vi "Habid_2-D_Histogram_Alpha.vi"() -> ()   [LabVIEW 2009]
uses:
  <vilib>/Utility/file.llb/Write To Spreadsheet File (DBL).vi
  <vilib>/Analysis/3filter.llb/Butterworth Filter (DBL).vi
  <vilib>/Analysis/NI_AALBase.lvlib
  <vilib>/Analysis/NI_AALPro.lvlib
panel:
  in  "Save 2-D":bool
  in  "Result File Dir 2":path
  in  "Result File Name 2":string="2D_Histogram.txt"
  in  "Piezo Factor":dbl=0.88881
  in  "High Voltage Gain":dbl=0.796905
  out "Total 2D Histogram":dbl[][](graph)
  out "Individual 2D Histogram":dbl[][](graph)
  out "After I(t)":cluster{dbl, dbl, "Filtered X":dbl[]}(graph)
  out "Before I(t)":cluster{dbl, "SamplingTime":dbl, "Data":ext[]}(graph)
  in  "start path":path=path "J:/data"
  out "NormAC":dbl[](array[numeric])
  in  "Save Curve?":bool
  out "CurrentFileName":string
  in  "Result File Name":string="1D_Histogram.txt"
  in  "Result File Dir":path
  in  "Save 1-D":bool
  out "SelectedCurves":i32
  out "CurvesInHistogram":bool[](array[boolean])
  in  "Bias(V)":dbl=0.4
  in  "Preamp(A/V)":dbl=1e-08
  out "1-D Histogram":cluster{dbl[], dbl[]}(graph)
  in  "Beta Cutoff max":dbl=20.0
  in  "Beta Cutoff min":dbl
  in  "1-D Histogram?":bool
  in  "Continuous?":bool
  in  "Add Histogram?":bool
  in  "Beta bins":i32=400
  in  "Beta max":dbl=20.0
  in  "Beta min":dbl
  in  "log(I) bins":i32=400
  in  "log(I) max":dbl=1.0
  in  "log(I) min":dbl=-3.0
  in  "+/-":bool=TRUE
  out "DcData":dbl[](array[numeric])
  out "Beta":dbl[](array[numeric])
  out "DcDataLog":dbl[](array[numeric])
  out "TotalCurves":i32
  out "CurrentCurve":i32
  in  "Next Curve":bool
  in  "Previous Curve":bool
  out "AC I(t)":T1(graph)
  in  "Piezo Sensitivity (nm/V)":dbl=3.89
  in  "Z-mod Amp (V)":dbl=0.0257
  in  "Gac/Gdc":dbl=1.43369
  in  "low cutoff freq: fl":u32=1200
  in  "high cutoff freq: fh":u32=2800
  out "DC I(t)":T2(graph)
  in  "DC cutoff freq":i32=600
  out "Original I(t)":cluster{dbl, "SamplingTime":dbl, "Data":ext[]}(graph)
  out "DataBuffer":dbl[](array[numeric])
  out "Sampling Freq":dbl
  out "Sampling Time":dbl
  out "TimeLine":dbl[](array[numeric])
  in  "stop":bool
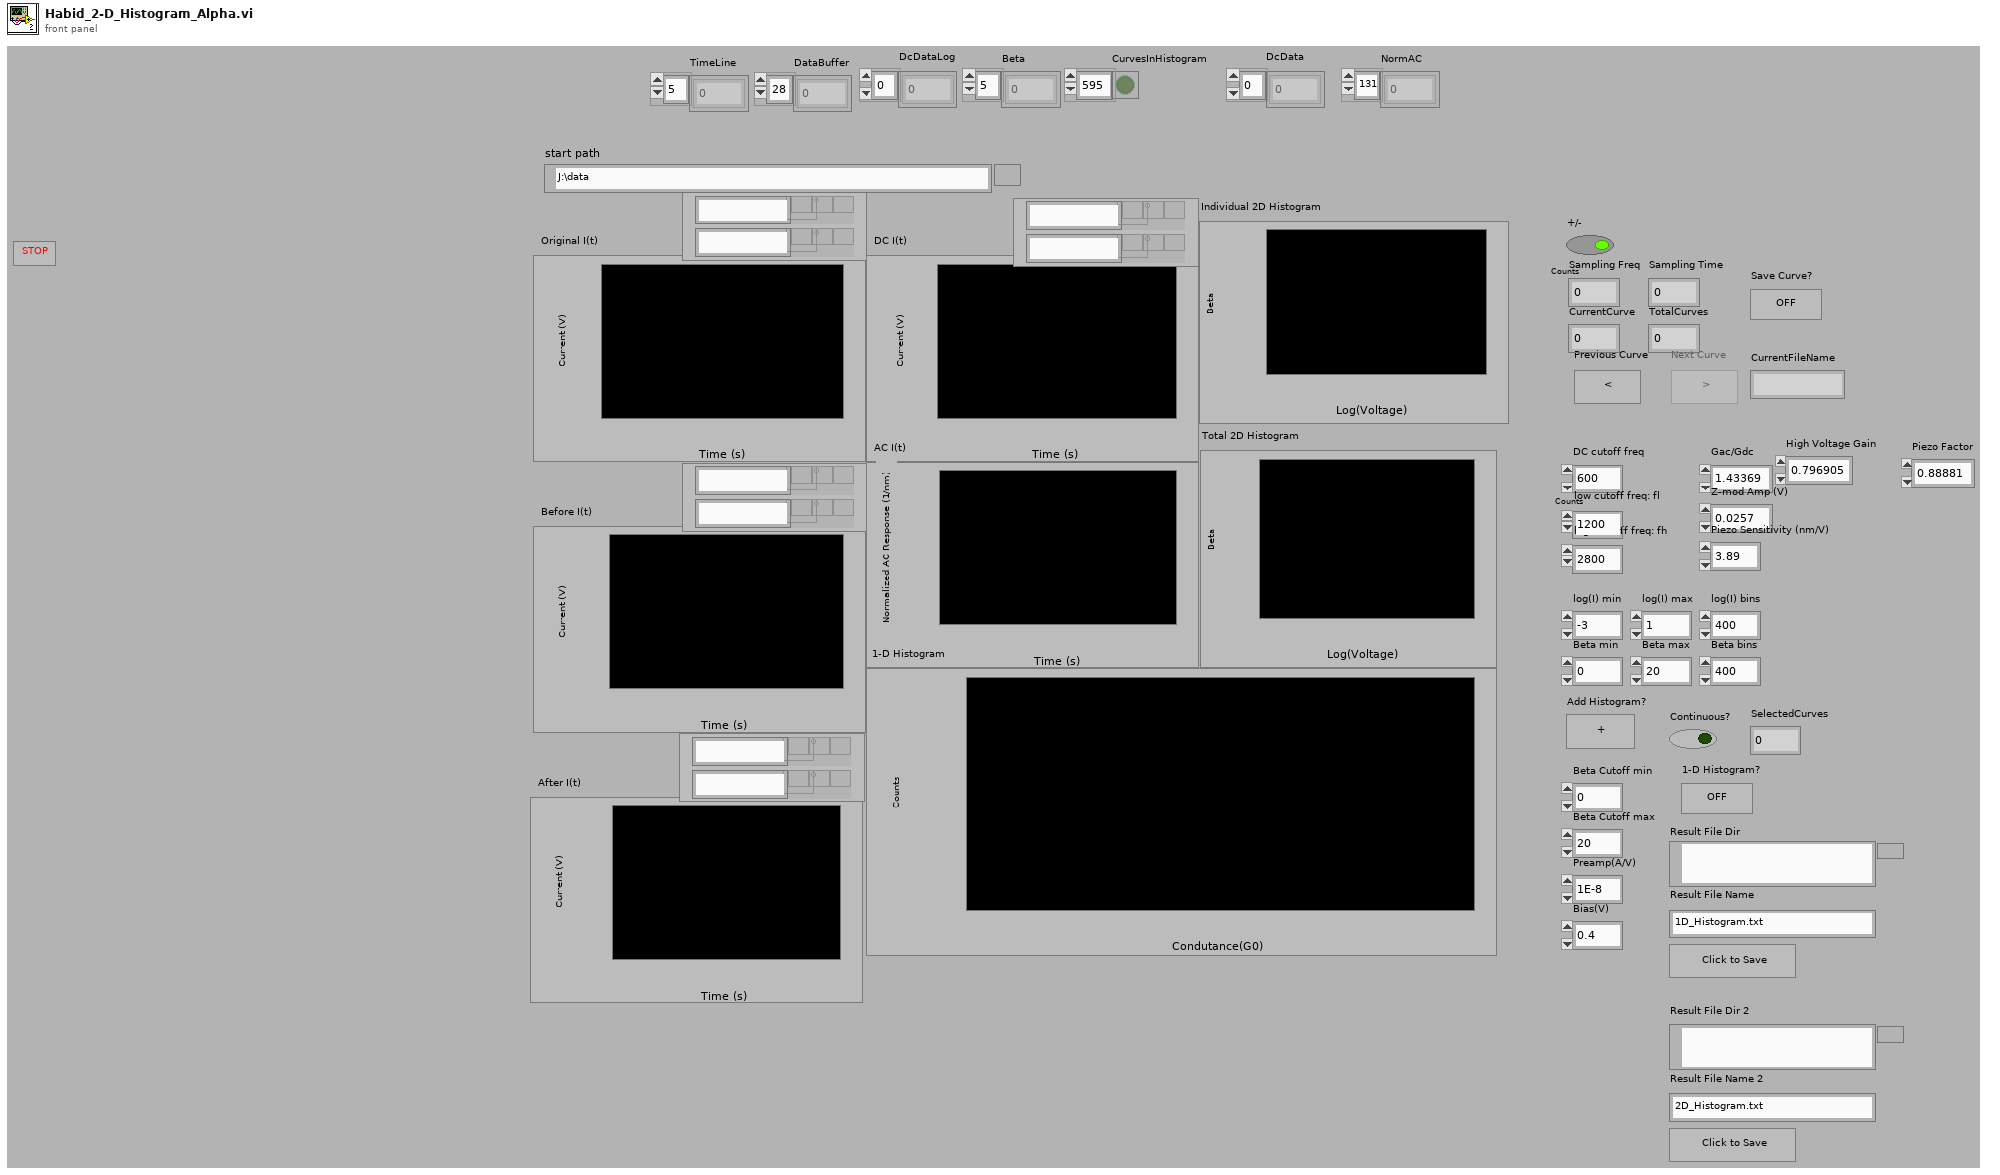
[diagram p1: front panel]
types:
  T1 = cluster{"Start Time":dbl, "Sampling Time":dbl, dbl[][]}
  T2 = cluster{dbl, "SamplingTime":dbl, "Filtered X":dbl[]}
  T3 = enum32{"Lowpass", "Highpass", "Bandpass", "Bandstop"}
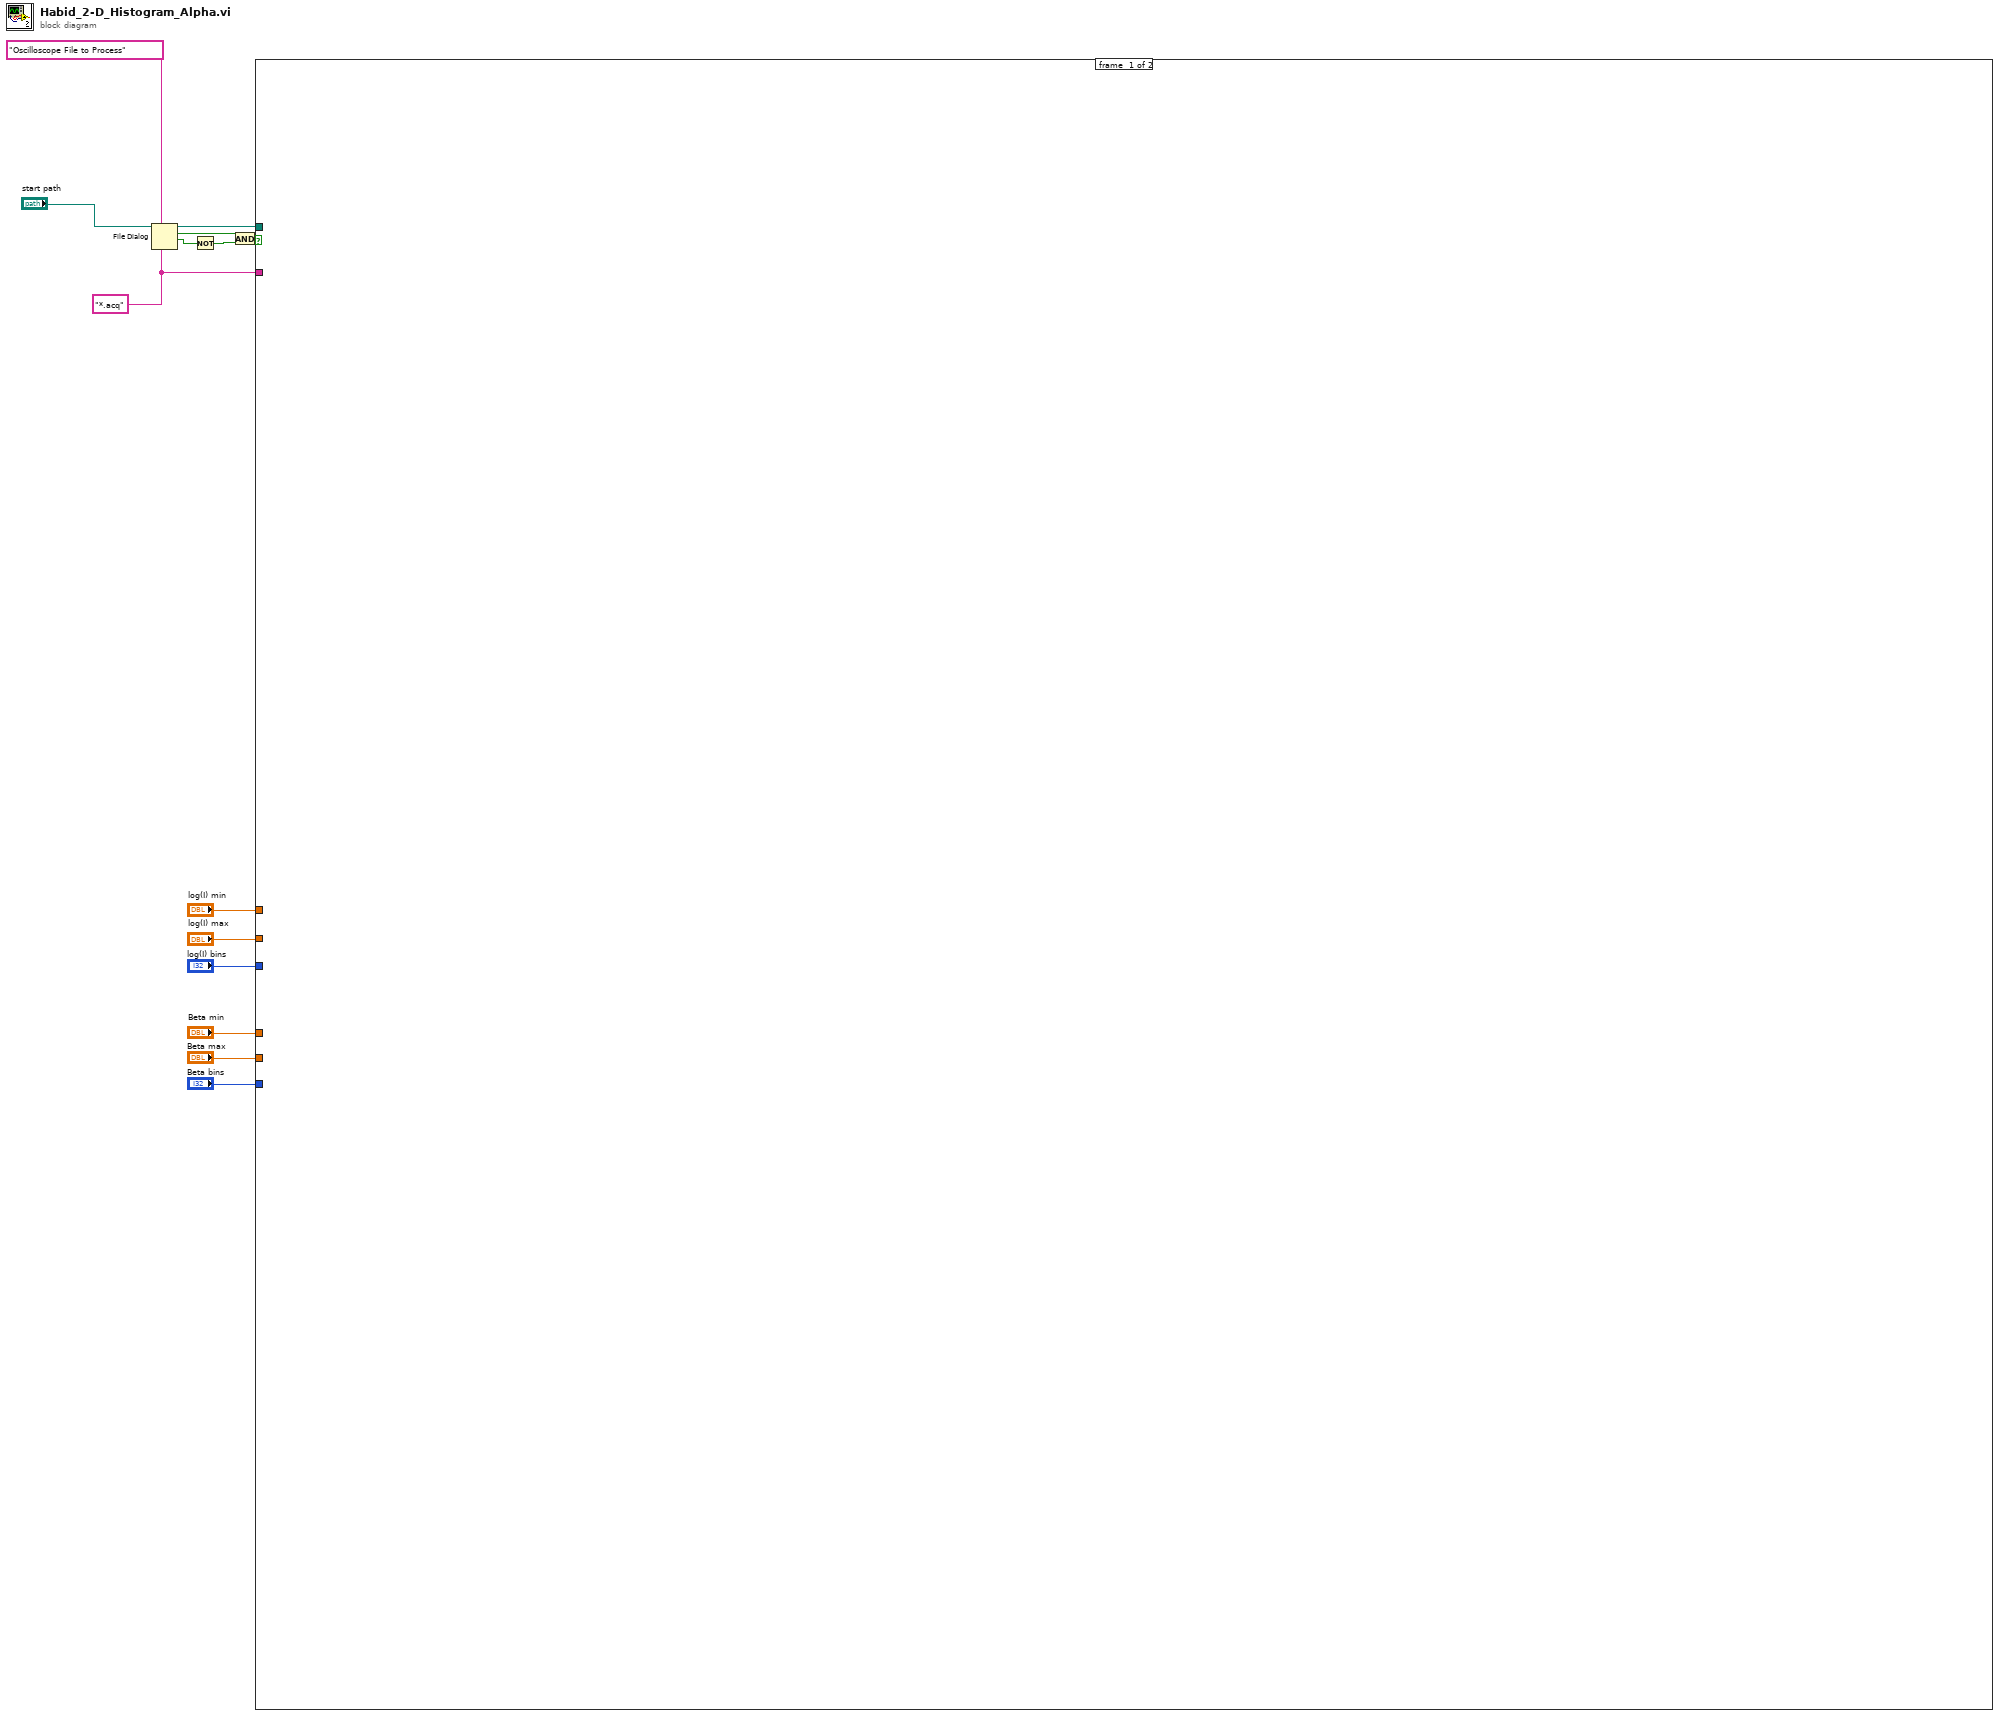
[diagram p0: block diagram]
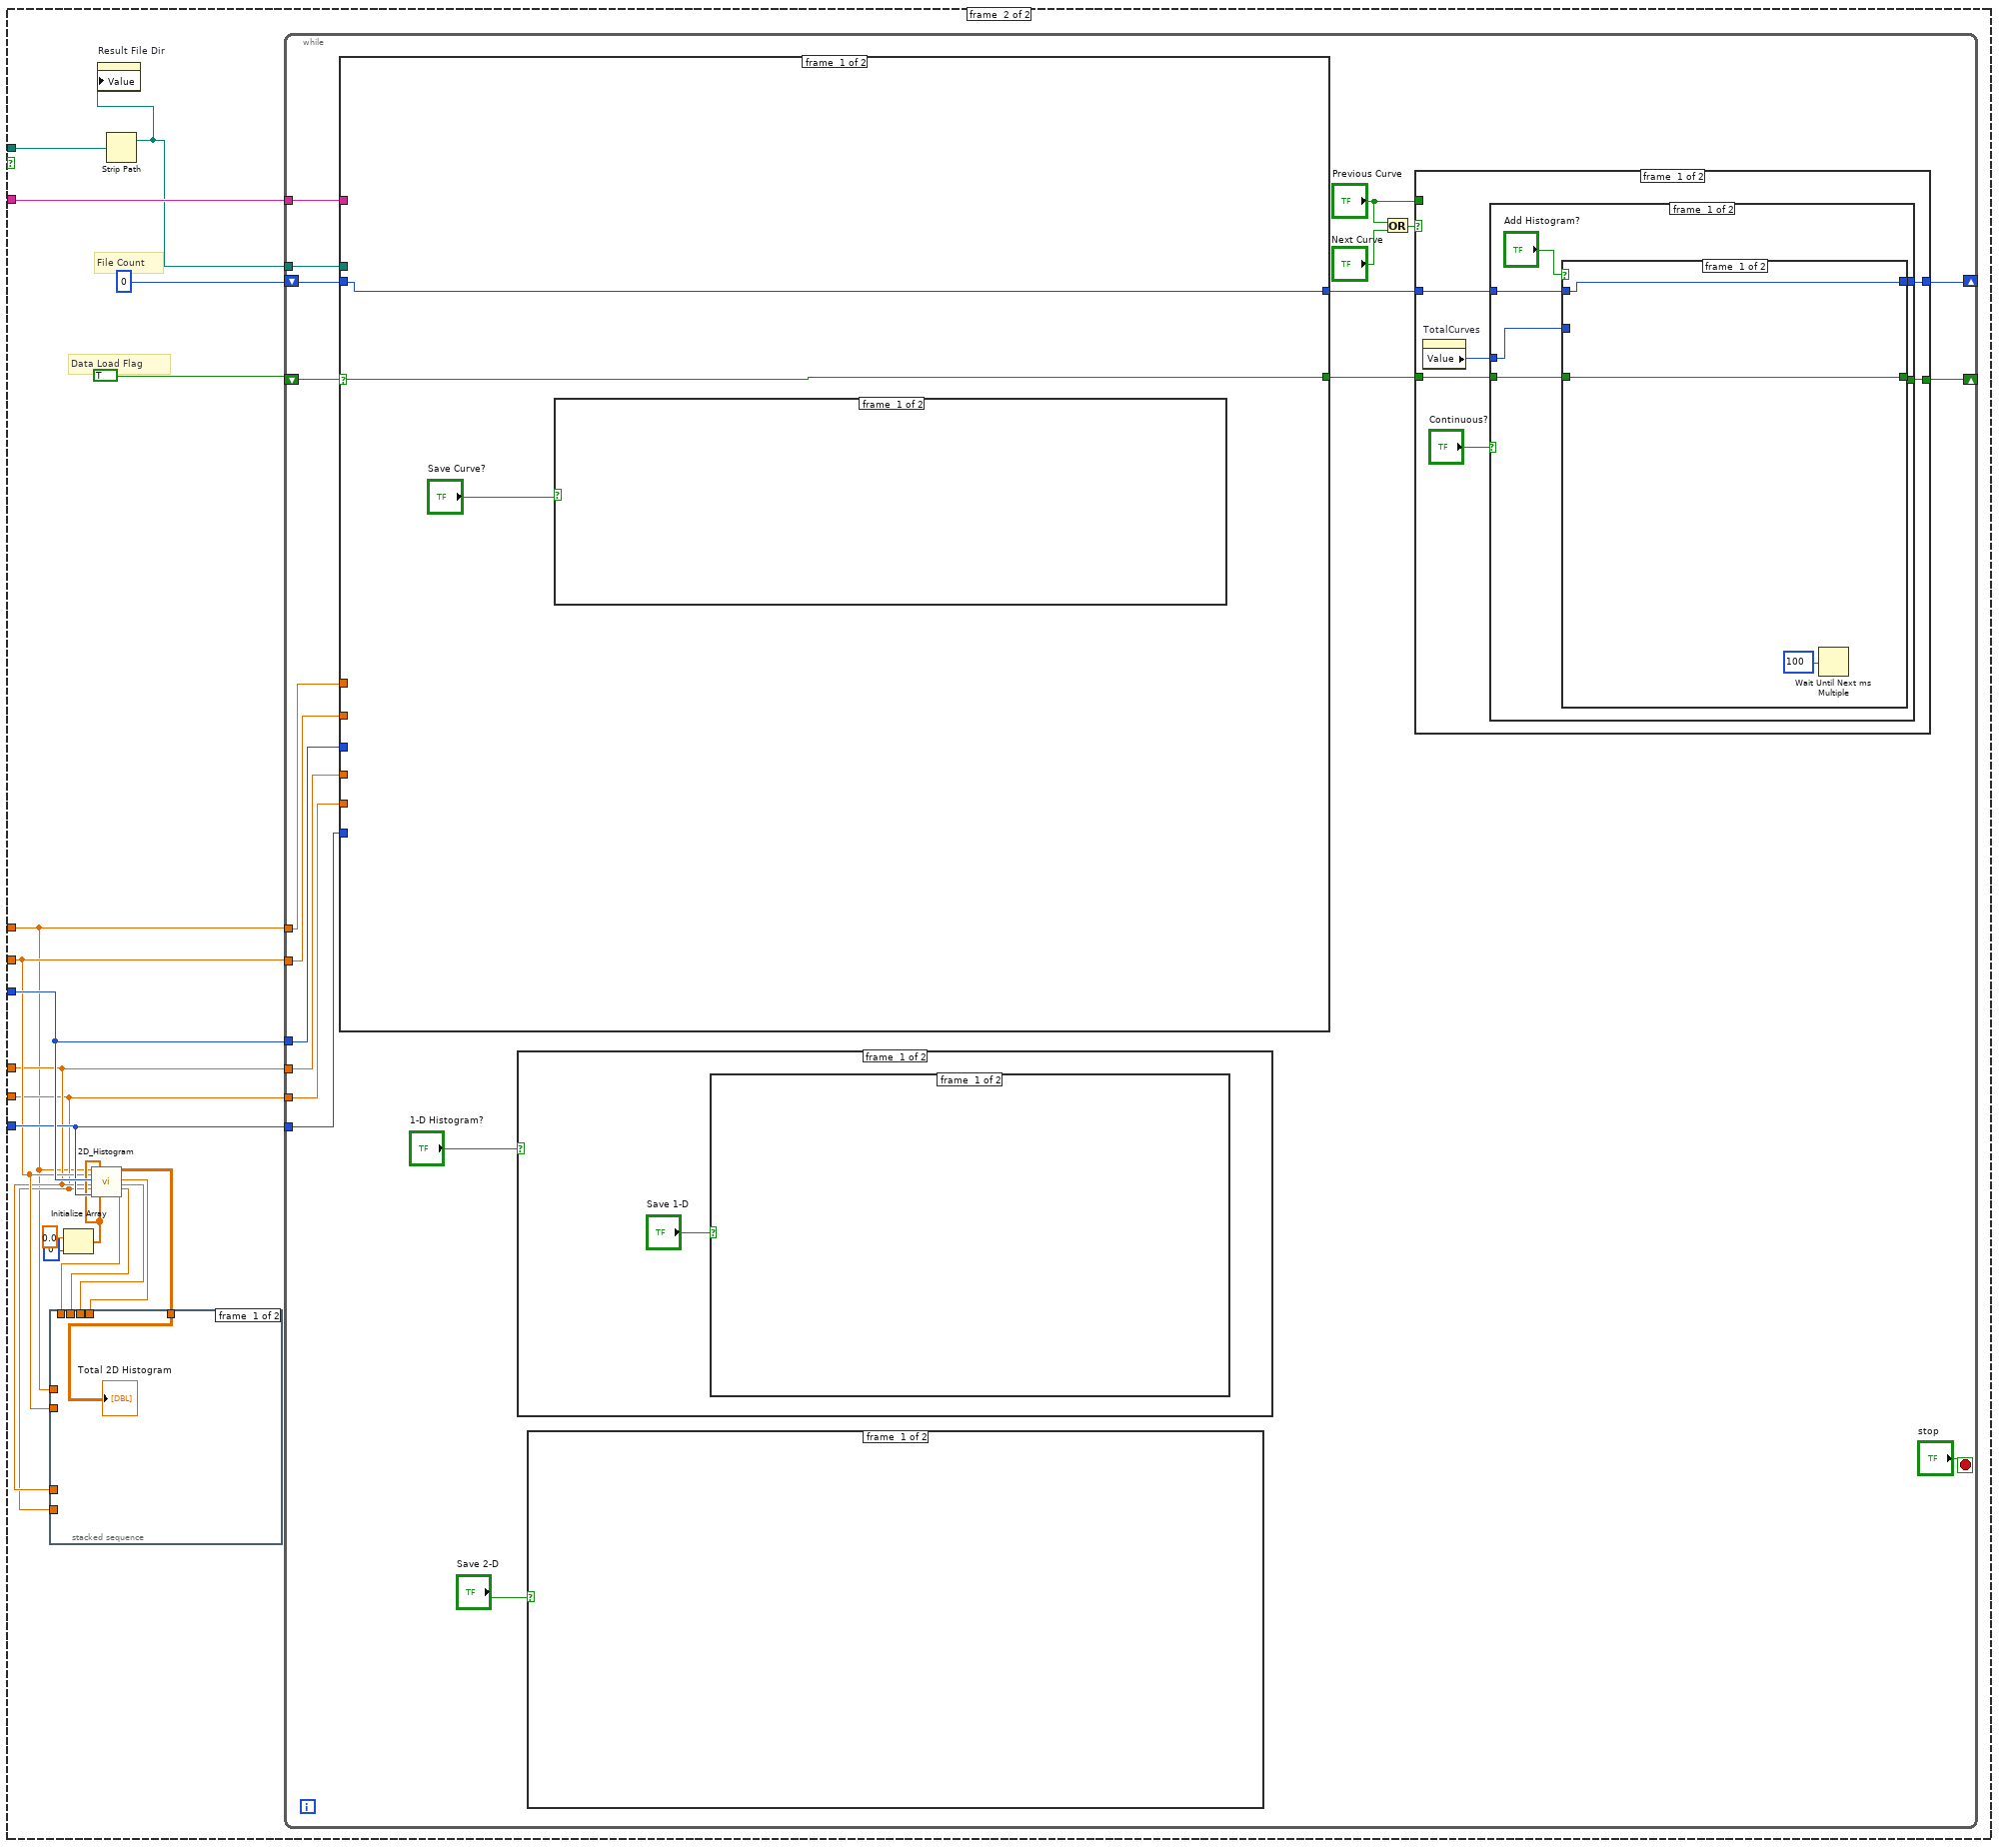
[diagram p2: hidden frame]
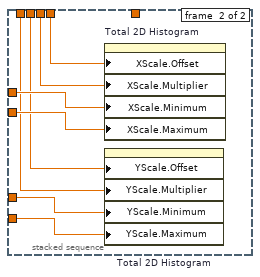
[diagram p3: hidden frame]
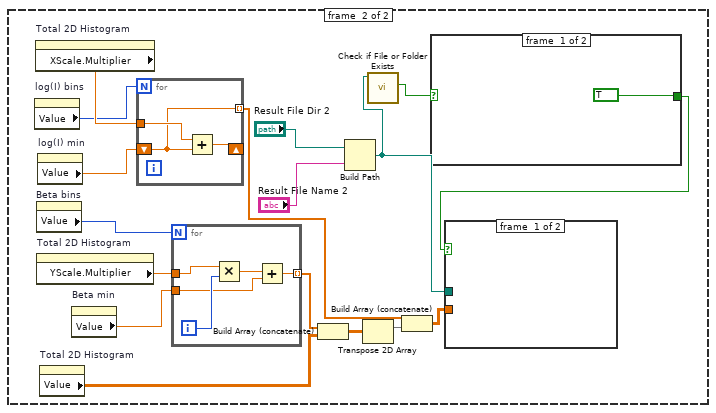
[diagram p4: hidden frame]
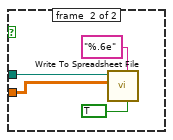
[diagram p5: hidden frame]
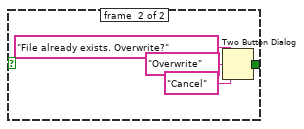
[diagram p6: hidden frame]
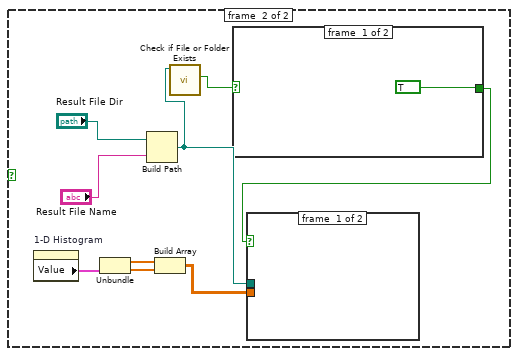
[diagram p7: hidden frame]
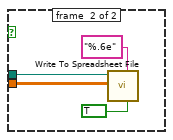
[diagram p8: hidden frame]
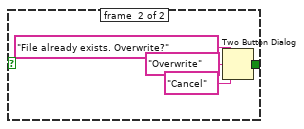
[diagram p9: hidden frame]
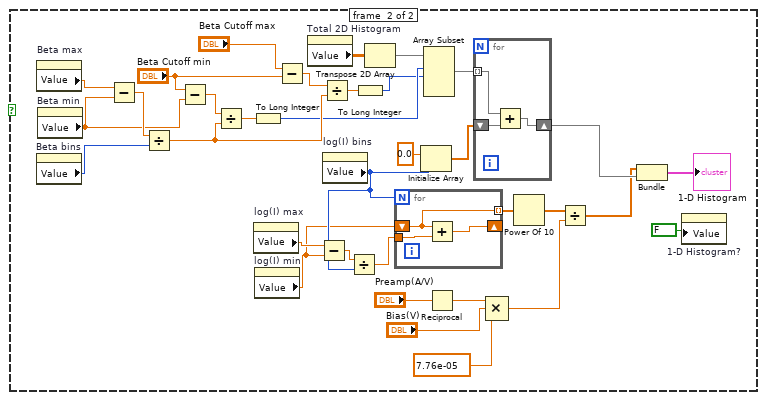
[diagram p10: hidden frame]
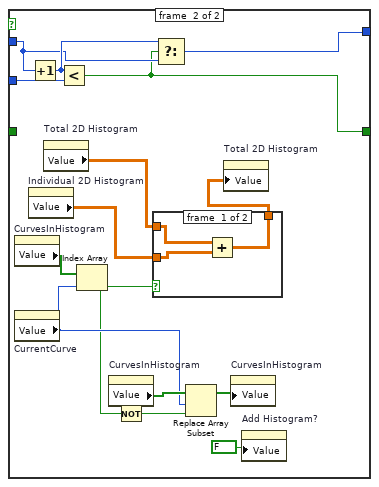
[diagram p11: hidden frame]
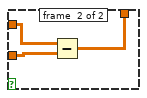
[diagram p12: hidden frame]
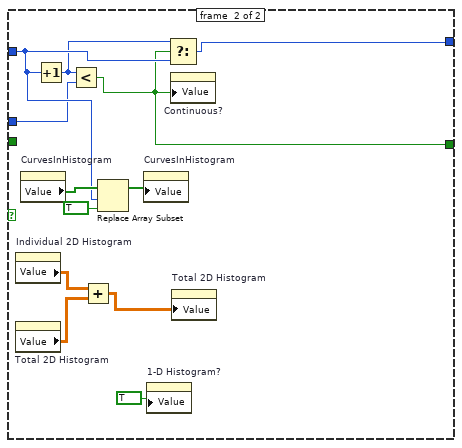
[diagram p13: hidden frame]
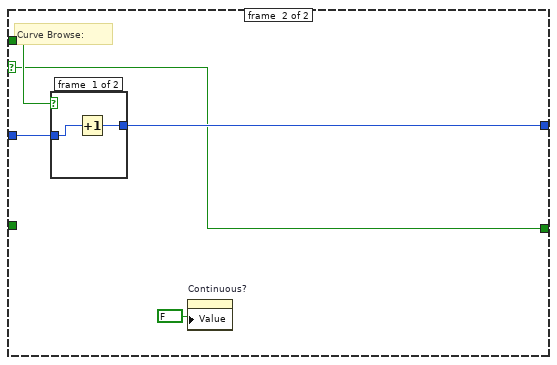
[diagram p14: hidden frame]
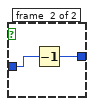
[diagram p15: hidden frame]
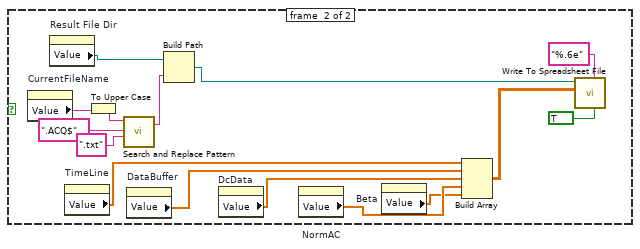
[diagram p16: hidden frame]
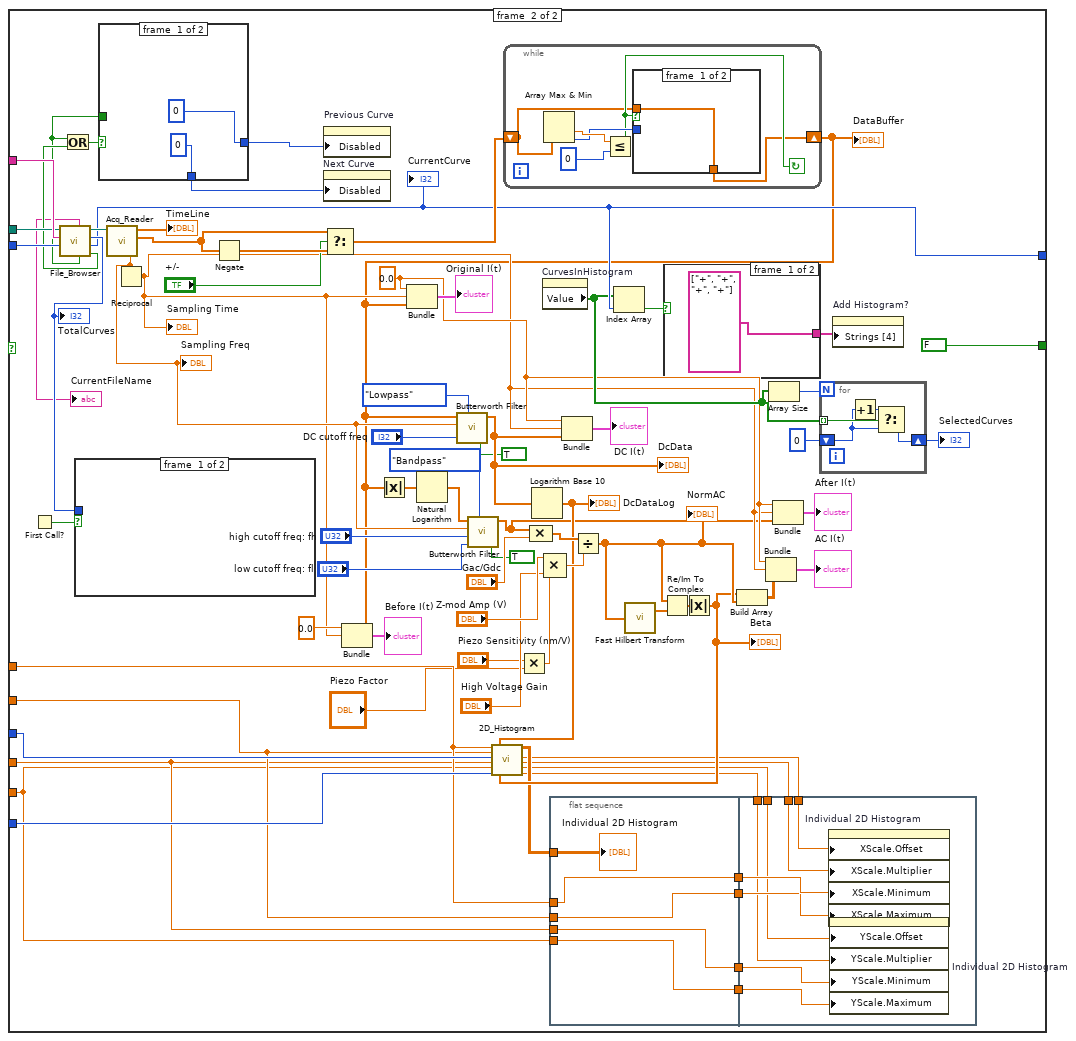
[diagram p17: hidden frame]
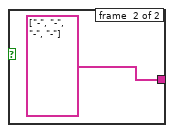
[diagram p18: hidden frame]
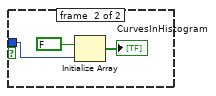
[diagram p19: hidden frame]
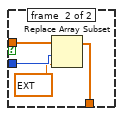
[diagram p20: hidden frame]
diagram:
  w7 = "*.acq" ("pattern (all files)")
  n1 = File Dialog(6:w7, 7:"Oscilloscope File to Process", 11:"start path") -> (1:w11:bool, 2:w13:bool, 3:w8:path)  [unwired: 4 in, 1 out]
  n2 = Not(x=w11) -> (.not. x?=w12:bool)
  n3 = And(x=w13, y=w12) -> (x .and. y?=w9:bool)
  n4 = case shown="True" w9 {
    tunnel: w8 -> [_ w33]
    tunnel: w7 -> [_ w31]
    tunnel: "log(I) min" -> [_ w15]
    tunnel: "log(I) max" -> [_ w18]
    tunnel: "log(I) bins" -> [_ w29]
    tunnel: "Beta min" -> [_ w17]
    tunnel: "Beta max" -> [_ w16]
    tunnel: "Beta bins" -> [_ w28]
    frame #0 {
    }
    frame #1 {
      # "File Count"
      # "Data Load Flag"
      n5 = Initialize Array(0.0 ("element"), 0 ("dimension size")) -> (w20:dbl[])
      n6 = call "2D_Histogram.vi"("X min"=w15, "X max"=w18, "X bins"=w29, "Y min"=w17, "Y max"=w16, "Y bins"=w28, "X"=w20, "Y"=w20) -> ("X-Y 2-D Histogram"=w27:dbl[][], "Xoffset"=w26:dbl, "Xmultiplier"=w25:dbl, "Yoffset"=w24:dbl, "Ymultiplier"=w23:dbl)  [unwired: 7 in]
      n7 = stacked-sequence {
        tunnel: w27 -> [w34 _]
        tunnel: w25 -> [_ w41]
        tunnel: w23 -> [_ w37]
        tunnel: w26 -> [_ w42]
        tunnel: w24 -> [_ w38]
        tunnel: w15 -> [_ w40]
        tunnel: w18 -> [_ w39]
        tunnel: w17 -> [_ w36]
        tunnel: w16 -> [_ w35]
        frame #0 {
          "Total 2D Histogram" <- w34
        }
        frame #1 {
          n8 = property on="Total 2D Histogram" class="IntGraph (strict)"("XScale.Offset"=w42, "XScale.Multiplier"=w41, "XScale.Minimum"=w40, "XScale.Maximum"=w39) -> ()  [unwired: 2 in, 2 out]
          n9 = property on="Total 2D Histogram" class="IntGraph (strict)"("YScale.Offset"=w38, "YScale.Multiplier"=w37, "YScale.Minimum"=w36, "YScale.Maximum"=w35) -> ()  [unwired: 2 in, 2 out]
        }
      }
      n10 = Strip Path(path=w33) -> (stripped path=w19:path)  [unwired: 1 out]
      n11 = property on="Result File Dir" class="Path"("Value"=w19) -> ()  [unwired: 2 in, 2 out]
      n12 = while {
        shift-right: [w45] -> _
        shift-left: TRUE ("DataReload") -> [w61]
        tunnel: w31 -> [w60]
        tunnel: w19 -> [w59]
        shift-right: [w46] -> _
        shift-left: 0 -> [w58]
        tunnel: w15 -> [w55]
        tunnel: w18 -> [w54]
        tunnel: w29 -> [w53]
        tunnel: w17 -> [w52]
        tunnel: w16 -> [w51]
        tunnel: w28 -> [w50]
        stop <- "stop" stop-if-true
        n13 = case shown="True" w61 {
          selector: w61 -> [w215 _]
          tunnel: w60 -> [_ w305]
          tunnel: w59 -> [_ w304]
          tunnel: w58 -> [w214 w303]
          tunnel: [w215 FALSE] -> w57
          tunnel: [w214 w259] -> w56
          tunnel: w55 -> [_ w254]
          tunnel: w54 -> [_ w253]
          tunnel: w53 -> [_ w265]
          tunnel: w52 -> [_ w252]
          tunnel: w51 -> [_ w251]
          tunnel: w50 -> [_ w264]
          frame #0 {
            n14 = case shown="True" "Save Curve?" {
              frame #0 {
              }
              frame #1 {
                n15 = property on="CurrentFileName" class="Str"() -> ("Value"=w226:string)  [unwired: 2 in, 2 out]
                n16 = property on="Result File Dir" class="Path"() -> ("Value"=w230:path)  [unwired: 2 in, 2 out]
                n17 = property on="TimeLine" class="Arr (strict)"() -> ("Value"=w220:dbl[])  [unwired: 2 in, 2 out]
                n18 = To Upper Case(1:w226) -> (0:w227:string)
                n19 = call <vilib>:"Search and Replace Pattern.vi"("string"=w227, "regular expression (\"\")"=".ACQ$" ("regular expression (\"\")"), "replace string (\"\")"=".txt" ("replace string (\"\")")) -> ("result string"=w225:string)  [unwired: 2 in, 1 out]
                n20 = property on="DataBuffer" class="Arr (strict)"() -> ("Value"=w219:dbl[])  [unwired: 2 in, 2 out]
                n21 = Build Path(base path=w230, name or relative path=w225) -> (appended path=w222:path)
                n22 = property on="DcData" class="Arr (strict)"() -> ("Value"=w218:dbl[])  [unwired: 2 in, 2 out]
                n23 = property on="NormAC" class="Arr (strict)"() -> ("Value"=w217:dbl[])  [unwired: 2 in, 2 out]
                n24 = property on="Beta" class="Arr (strict)"() -> ("Value"=w216:dbl[])  [unwired: 2 in, 2 out]
                n25 = Build Array(w220, w219, w218, w217, w216) -> (w221:dbl[][])
                n26 = call-poly <vilib>:"Write To Spreadsheet File.vi"("transpose? (no:F)"=TRUE, "format (%.3f)"="%.6e", "2D data"=w221, "file path (dialog if empty)"=w222) -> ()  [unwired: 4 in, 1 out]
              }
            }
          }
          frame #1 {
            w240 = 0.0
            n27 = First Call?() -> (First Call?: T/F=w263:bool)
            n28 = call "File_Browser.vi"("FileIndexIn"=w303, "FileExt"=w305, "FolderPath"=w304) -> ("Last?"=w280:bool, "FileIndexOut"=w259:i32, "FileTotal"=w262:i32, "FullFilePath"=w302:path, "First?"=w279:bool, "FileName"=→"CurrentFileName":string)  [unwired: 3 in]
            "CurrentCurve" <- w259
            "TotalCurves" <- w262
            n29 = Or(x=w279, y=w280) -> (x .or. y?=w283:bool)
            n30 = case shown="True" w263 {
              tunnel: w262 -> [_ w313]
              frame #0 {
              }
              frame #1 {
                n31 = Initialize Array(FALSE ("DataReload"), w313) -> (→"CurvesInHistogram":bool[])
              }
            }
            n32 = case shown="True" w283 {
              tunnel: w279 -> [_ w343]
              tunnel: [0 w342] -> w281
              tunnel: [0 w341] -> w282
              frame #0 {
              }
              frame #1 {
                # "Button Control:"
                n33 = case shown="True" w343 {
                  tunnel: [0 2] -> w342
                  tunnel: [2 0] -> w341
                  frame #0 {
                  }
                  frame #1 {
                  }
                }
              }
            }
            n34 = call "Acq_Reader.vi"("AcqFileToRead"=w302) -> ("SamplingFreq"=w278:dbl, "Data"=w275:ext[], "TimeLine"=→"TimeLine":dbl[])  [unwired: 8 in]
            "Sampling Freq" <- w278
            n35 = Reciprocal(x=w278) -> (1/x=w239:dbl)
            "Sampling Time" <- w239
            n36 = Negate(x=w275) -> (-x=w274:ext[])
            n37 = property on="Previous Curve" class="Bool"("Disabled"=w281) -> ()  [unwired: 2 in, 2 out]
            n38 = property on="Next Curve" class="Bool"("Disabled"=w282) -> ()  [unwired: 2 in, 2 out]
            n39 = Select(t=w275, s="+/-", f=w274) -> (s? t:f=w276:ext[])
            n40 = while {
              shift-right: [w328] -> w233
              shift-left: w276 -> [w329]
              stop <- w330 continue-if-true
              n41 = Array Max & Min(array=w329) -> (min value=w332:ext, min index (indices)=w331:i32)  [unwired: 2 out]
              n42 = Less Or Equal?(x=w332, y=0) -> (x <= y?=w330:bool)
              n43 = case shown="True" w330 {
                tunnel: w331 -> [_ w338]
                tunnel: w329 -> [w334 w337]
                tunnel: [w334 w336] -> w328
                frame #0 {
                }
                frame #1 {
                  n44 = Replace Array Subset(array=w337, new element=ext 0.00000100000000000000000004 ("new element/subarray"), index=w338) -> (w336:ext[])
                }
              }
            }
            "DataBuffer" <- w233
            n45 = Bundle(0.0, w239, "Data"=w233) -> (→"Before I(t)":cluster{dbl, dbl, "Data":ext[]})  [unwired: 1 in]
            n46 = Absolute Value(x=w233) -> (abs(x)=w232:ext[])
            n47 = Bundle(w240, w239, "Data"=w233) -> (→"Original I(t)":cluster{dbl, dbl, "Data":ext[]})  [unwired: 1 in]
            n48 = Natural Logarithm(1:w232) -> (0:w231:ext[])
            n49 = call-poly <vilib>:"Butterworth Filter.vi"("init/cont (init:F)"=TRUE, "filter type"=T3."Lowpass", "low cutoff freq: fl"="DC cutoff freq", "sampling freq: fs"=w278, "X"=w233) -> ("Filtered X"=w277:dbl[])  [unwired: 3 in, 1 out]
            "DcData" <- w277
            n50 = call-poly <vilib>:"Butterworth Filter.vi"("init/cont (init:F)"=TRUE, "filter type"=T3."Bandpass", "low cutoff freq: fl"="low cutoff freq: fl", "high cutoff freq: fh"="high cutoff freq: fh", "sampling freq: fs"=w278, "X"=w231) -> ("Filtered X"=w238:dbl[])  [unwired: 2 in, 1 out]
            n51 = Multiply(x="Piezo Sensitivity (nm/V)", y="Piezo Factor") -> (x*y=w236:dbl)
            n52 = Compound Arithmetic op=MULTIPLY(w238, "Gac/Gdc") -> (w291:dbl[])
            n53 = Logarithm Base 10(1:w277) -> (0:w272:dbl[])
            "DcDataLog" <- w272
            n54 = property on="CurvesInHistogram" class="Arr (strict)"() -> ("Value"=w256:bool[])  [unwired: 2 in, 2 out]
            n55 = Compound Arithmetic op=MULTIPLY("Z-mod Amp (V)", w236, "High Voltage Gain") -> (w290:dbl)
            n56 = flat-sequence {
              tunnel: w270 -> [w315]
              tunnel: w254 -> [w319]
              tunnel: w253 -> [w318]
              tunnel: w252 -> [w317]
              tunnel: w251 -> [w316]
              tunnel: [w319] -> w250
              tunnel: [w318] -> w249
              tunnel: [w317] -> w248
              tunnel: [w316] -> w247
              tunnel: w269 -> [w326]
              tunnel: w268 -> [w322]
              tunnel: w267 -> [w327]
              tunnel: w266 -> [w323]
              tunnel: w250 -> [w325]
              tunnel: w249 -> [w324]
              tunnel: w248 -> [w321]
              tunnel: w247 -> [w320]
              frame #0 {
                "Individual 2D Histogram" <- w315
              }
              frame #1 {
                n57 = property on="Individual 2D Histogram" class="IntGraph (strict)"("XScale.Offset"=w327, "XScale.Multiplier"=w326, "XScale.Minimum"=w325, "XScale.Maximum"=w324) -> ()  [unwired: 2 in, 2 out]
                n58 = property on="Individual 2D Histogram" class="IntGraph (strict)"("YScale.Offset"=w323, "YScale.Multiplier"=w322, "YScale.Minimum"=w321, "YScale.Maximum"=w320) -> ()  [unwired: 2 in, 2 out]
              }
            }
            n59 = Bundle(w240, w239, "Filtered X"=w277) -> (→"DC I(t)":cluster{dbl, dbl, "Filtered X":dbl[]})  [unwired: 1 in]
            n60 = Divide(x=w291, y=w290) -> (x/y=w285:dbl[])
            "NormAC" <- w285
            n61 = Index Array(array=w256, index=w259) -> (element=w261:bool)
            n62 = call <vilib>:"Fast Hilbert Transform.vi"("X"=w285) -> ("Hilbert{X}"=w289:dbl[])  [unwired: 1 out]
            n63 = Re/Im To Complex(1:w289, 2:w285) -> (0:w288:cdb[])
            n64 = case shown="False" w261 {
              tunnel: [string[] ["+", "+", "+", "+"] ("Strings [4]") string[] ["-", "-", "-", "-"] ("Strings [4]")] -> w260
              frame #0 {
              }
              frame #1 {
              }
            }
            n65 = Absolute Value(x=w288) -> (abs(x)=w271:dbl[])
            "Beta" <- w271
            n66 = call "2D_Histogram.vi"("X min"=w254, "X max"=w253, "X bins"=w265, "Y min"=w252, "Y max"=w251, "Y bins"=w264, "X"=w272, "Y"=w271) -> ("X-Y 2-D Histogram"=w270:dbl[][], "Xoffset"=w267:dbl, "Xmultiplier"=w269:dbl, "Yoffset"=w266:dbl, "Ymultiplier"=w268:dbl)  [unwired: 7 in]
            n67 = Build Array(w271, w285) -> (w287:dbl[][])
            n68 = Bundle(w240, w239, w287) -> (→"AC I(t)":cluster{dbl, dbl, dbl[][]})  [unwired: 1 in]
            n69 = Array Size(array=w256) -> (size(s)=w258:i32)
            n70 = Bundle(w240, w239, "Filtered X"=w238) -> (→"After I(t)":cluster{dbl, dbl, "Filtered X":dbl[]})  [unwired: 1 in]
            n71 = for {
              N: w258 -> [_]
              shift-right: [w306] -> w255
              shift-left: 0 -> [w308]
              tunnel: w256 -> [w309] mode=indexing
              n72 = Increment(x=w308) -> (x+1=w307:i32)
              n73 = Select(t=w307, s=w309, f=w308) -> (s? t:f=w306:i32)
            }
            "SelectedCurves" <- w255
            n74 = property on="Add Histogram?" class="Bool (strict)"("Strings [4]"=w260) -> ()  [unwired: 2 in, 2 out]
          }
        }
        n75 = case shown="True" "1-D Histogram?" {
          frame #0 {
            n76 = case shown="True" "Save 1-D" {
              frame #0 {
              }
              frame #1 {
                n77 = property on="1-D Histogram" class="XYGraph (strict)"() -> ("Value"=w106:cluster{dbl[], dbl[]})  [unwired: 2 in, 2 out]
                n78 = Unbundle(w106) -> (w105:dbl[], w104:dbl[])
                n79 = Build Path(base path="Result File Dir", name or relative path="Result File Name") -> (appended path=w99:path)
                n80 = Build Array(w105, w104) -> (w98:dbl[][])
                n81 = call <vilib>:"Check if File or Folder Exists.vi"("path"=w99) -> ("file or folder exists?"=w101:bool)  [unwired: 8 in, 2 out]
                n82 = case shown="True" w101 {
                  tunnel: [TRUE ("T button?") w112] -> w100
                  frame #0 {
                  }
                  frame #1 {
                    n83 = Two Button Dialog(message="File already exists. Overwrite?", 1:"Cancel" ("F button name (\"Cancel\")"), 2:"Overwrite" ("T button name (\"OK\")")) -> (T button?=w112:bool)
                  }
                }
                n84 = case shown="True" w100 {
                  tunnel: w98 -> [_ w108]
                  tunnel: w99 -> [_ w109]
                  frame #0 {
                  }
                  frame #1 {
                    n85 = call-poly <vilib>:"Write To Spreadsheet File.vi"("transpose? (no:F)"=TRUE, "format (%.3f)"="%.6e", "2D data"=w108, "file path (dialog if empty)"=w109) -> ()  [unwired: 4 in, 1 out]
                  }
                }
              }
            }
          }
          frame #1 {
            n86 = property on="Beta max" class="DigNum (strict)"() -> ("Value"=w149:dbl)  [unwired: 2 in, 2 out]
            n87 = property on="Beta bins" class="DigNum (strict)"() -> ("Value"=w147:i32)  [unwired: 2 in, 2 out]
            n88 = property on="Beta min" class="DigNum (strict)"() -> ("Value"=w146:dbl)  [unwired: 2 in, 2 out]
            n89 = Subtract(x=w149, y=w146) -> (x-y=w148:dbl)
            n90 = Divide(x=w148, y=w147) -> (x/y=w140:dbl)
            n91 = Subtract(x="Beta Cutoff min", y=w146) -> (x-y=w145:dbl)
            n92 = Divide(x=w145, y=w140) -> (x/y=w144:dbl)
            n93 = To Long Integer(number=w144) -> (32bit integer=w138:i32)
            n94 = property on="log(I) max" class="DigNum (strict)"() -> ("Value"=w128:dbl)  [unwired: 2 in, 2 out]
            n95 = property on="log(I) min" class="DigNum (strict)"() -> ("Value"=w119:dbl)  [unwired: 2 in, 2 out]
            n96 = Subtract(x="Beta Cutoff max", y="Beta Cutoff min") -> (x-y=w141:dbl)
            n97 = property on="Total 2D Histogram" class="IntGraph (strict)"() -> ("Value"=w116:dbl[][])  [unwired: 2 in, 2 out]
            n98 = Subtract(x=w128, y=w119) -> (x-y=w132:dbl)
            n99 = Divide(x=w141, y=w140) -> (x/y=w139:dbl)
            n100 = property on="log(I) bins" class="DigNum (strict)"() -> ("Value"=w129:i32)  [unwired: 2 in, 2 out]
            n101 = Divide(x=w132, y=w129) -> (x/y=w127:dbl)
            n102 = To Long Integer(number=w139) -> (32bit integer=w137:i32)
            n103 = Transpose 2D Array(2D array=w116) -> (transposed array=w130:dbl[][])
            n104 = for {
              N: w129 -> [_]
              shift-right: [w152] -> _
              shift-left: w119 -> [w150]
              tunnel: w127 -> [w151]
              tunnel: [w150] -> w126 mode=indexing
              n105 = Add(x=w150, y=w151) -> (x+y=w152:dbl)
            }
            n106 = Initialize Array(0.0 ("element"), w129) -> (w134:dbl[])
            n107 = Array Subset(array=w130, index (row)=w138, length (row)=w137) -> (w135:dbl[][])  [unwired: 2 in]
            n108 = Reciprocal(x="Preamp(A/V)") -> (1/x=w121:dbl)
            n109 = for {
              tunnel: w135 -> [w155] mode=indexing
              shift-right: [w153] -> w133
              shift-left: w134 -> [w154]
              n110 = Add(x=w155, y=w154) -> (x+y=w153:dbl[])
            }
            n111 = Compound Arithmetic op=MULTIPLY(w121, "Bias(V)", 7.76e-05 ("value")) -> (w117:dbl)
            n112 = Power Of 10(x=w126) -> (10^x=w120:dbl[])
            n113 = Divide(x=w120, y=w117) -> (x/y=w118:dbl[])
            n114 = Bundle(w118, w133) -> (→"1-D Histogram":cluster{dbl[], dbl[]})  [unwired: 1 in]
            n115 = property on="1-D Histogram?" class="Bool (strict)"("Value"=FALSE ("1-D Histogram?")) -> ()  [unwired: 2 in, 2 out]
          }
        }
        n116 = case shown="True" "Save 2-D" {
          frame #0 {
          }
          frame #1 {
            n117 = property on="log(I) bins" class="DigNum (strict)"() -> ("Value"=w70:i32)  [unwired: 2 in, 2 out]
            n118 = property on="Total 2D Histogram" class="IntGraph (strict)"() -> ("XScale.Multiplier"=w71:dbl)  [unwired: 2 in, 2 out]
            n119 = property on="Beta bins" class="DigNum (strict)"() -> ("Value"=w74:i32)  [unwired: 2 in, 2 out]
            n120 = property on="Total 2D Histogram" class="IntGraph (strict)"() -> ("YScale.Multiplier"=w73:dbl)  [unwired: 2 in, 2 out]
            n121 = property on="log(I) min" class="DigNum (strict)"() -> ("Value"=w69:dbl)  [unwired: 2 in, 2 out]
            n122 = property on="Total 2D Histogram" class="IntGraph (strict)"() -> ("Value"=w68:dbl[][])  [unwired: 2 in, 2 out]
            n123 = property on="Beta min" class="DigNum (strict)"() -> ("Value"=w72:dbl)  [unwired: 2 in, 2 out]
            n124 = for {
              N: w70 -> [_]
              tunnel: w71 -> [w82]
              shift-right: [w81] -> _
              shift-left: w69 -> [w80]
              tunnel: [w80] -> w64 mode=indexing
              n125 = Add(x=w82, y=w80) -> (x+y=w81:dbl)
            }
            n126 = for {
              N: w74 -> [_]
              tunnel: w73 -> [w85]
              tunnel: w72 -> [w84]
              tunnel: [w83] -> w67 mode=indexing
              i -> [w86]
              n127 = Multiply(x=w85, y=w86) -> (x*y=w87:dbl)
              n128 = Add(x=w87, y=w84) -> (x+y=w83:dbl)
            }
            n129 = Build Array (concatenate)(w67, w68) -> (w66:dbl[][])
            n130 = Build Path(base path="Result File Dir 2", name or relative path="Result File Name 2") -> (appended path=w75:path)
            n131 = Transpose 2D Array(2D array=w66) -> (transposed array=w65:dbl[][])
            n132 = call <vilib>:"Check if File or Folder Exists.vi"("path"=w75) -> ("file or folder exists?"=w77:bool)  [unwired: 8 in, 2 out]
            n133 = Build Array (concatenate)(w64, w65) -> (w63:dbl[][])
            n134 = case shown="True" w77 {
              tunnel: [TRUE ("T button?") w93] -> w76
              frame #0 {
              }
              frame #1 {
                n135 = Two Button Dialog(message="File already exists. Overwrite?", 1:"Cancel" ("F button name (\"Cancel\")"), 2:"Overwrite" ("T button name (\"OK\")")) -> (T button?=w93:bool)
              }
            }
            n136 = case shown="True" w76 {
              tunnel: w75 -> [_ w90]
              tunnel: w63 -> [_ w88]
              frame #0 {
              }
              frame #1 {
                n137 = call-poly <vilib>:"Write To Spreadsheet File.vi"("transpose? (no:F)"=TRUE, "format (%.3f)"="%.6e", "2D data"=w88, "file path (dialog if empty)"=w90) -> ()  [unwired: 4 in, 1 out]
              }
            }
          }
        }
        n138 = Or(x="Previous Curve", y="Next Curve") -> (x .or. y?=w48:bool)
        n139 = case shown="False" w48 {
          selector: w48 -> [_ w205]
          tunnel: "Previous Curve" -> [_ w208]
          tunnel: w56 -> [w158 w207]
          tunnel: [w157 w206] -> w46
          tunnel: w57 -> [w161 _]
          tunnel: [w160 w205] -> w45
          frame #0 {
            n140 = property on="TotalCurves" class="DigNum (strict)"() -> ("Value"=w156:i32)  [unwired: 2 in, 2 out]
            n141 = case shown="False" "Continuous?" {
              tunnel: w161 -> [w164 _]
              tunnel: [w163 w195] -> w160
              tunnel: w158 -> [w166 w200]
              tunnel: [w165 w203] -> w157
              tunnel: w156 -> [w162 w197]
              frame #0 {
                n142 = case shown="True" "Add Histogram?" {
                  tunnel: w166 -> [w170 w176]
                  tunnel: [w170 w175] -> w165
                  tunnel: w164 -> [w169 _]
                  tunnel: [w169 w174] -> w163
                  tunnel: w162 -> [_ w178]
                  frame #0 {
                    n143 = Wait Until Next ms Multiple(millisecond multiple=u32 100) -> ()  [unwired: 1 out]
                  }
                  frame #1 {
                    n144 = property on="CurvesInHistogram" class="Arr (strict)"() -> ("Value"=w184:bool[])  [unwired: 2 in, 2 out]
                    n145 = property on="CurrentCurve" class="DigNum (strict)"() -> ("Value"=w181:i32)  [unwired: 2 in, 2 out]
                    n146 = property on="Individual 2D Histogram" class="IntGraph (strict)"() -> ("Value"=w173:dbl[][])  [unwired: 2 in, 2 out]
                    n147 = Increment(x=w176) -> (x+1=w177:i32)
                    n148 = property on="Total 2D Histogram" class="IntGraph (strict)"() -> ("Value"=w172:dbl[][])  [unwired: 2 in, 2 out]
                    n149 = Less?(x=w177, y=w178) -> (x < y?=w174:bool)
                    n150 = Index Array(array=w184, index=w181) -> (element=w180:bool)
                    n151 = property on="CurvesInHistogram" class="Arr (strict)"() -> ("Value"=w183:bool[])  [unwired: 2 in, 2 out]
                    n152 = Not(x=w180) -> (.not. x?=w179:bool)
                    n153 = case shown="True" w180 {
                      tunnel: w172 -> [w188 w191]
                      tunnel: w173 -> [w187 w190]
                      tunnel: [w186 w189] -> w171
                      frame #0 {
                        n154 = Add(x=w188, y=w187) -> (x+y=w186:dbl[][])
                      }
                      frame #1 {
                        n155 = Subtract(x=w191, y=w190) -> (x-y=w189:dbl[][])
                      }
                    }
                    n156 = Select(t=w177, s=w174, f=w176) -> (s? t:f=w175:i32)
                    n157 = Replace Array Subset(array=w183, new element=w179, index=w181) -> (w182:bool[])
                    n158 = property on="Total 2D Histogram" class="IntGraph (strict)"("Value"=w171) -> ()  [unwired: 2 in, 2 out]
                    n159 = property on="CurvesInHistogram" class="Arr (strict)"("Value"=w182) -> ()  [unwired: 2 in, 2 out]
                    n160 = property on="Add Histogram?" class="Bool (strict)"("Value"=FALSE ("Add Histogram?")) -> ()  [unwired: 2 in, 2 out]
                  }
                }
              }
              frame #1 {
                n161 = property on="Individual 2D Histogram" class="IntGraph (strict)"() -> ("Value"=w194:dbl[][])  [unwired: 2 in, 2 out]
                n162 = property on="Total 2D Histogram" class="IntGraph (strict)"() -> ("Value"=w192:dbl[][])  [unwired: 2 in, 2 out]
                n163 = property on="CurvesInHistogram" class="Arr (strict)"() -> ("Value"=w201:bool[])  [unwired: 2 in, 2 out]
                n164 = Increment(x=w200) -> (x+1=w196:i32)
                n165 = Less?(x=w196, y=w197) -> (x < y?=w195:bool)
                n166 = Add(x=w194, y=w192) -> (x+y=w193:dbl[][])
                n167 = Replace Array Subset(array=w201, new element=TRUE ("new element/subarray"), index=w200) -> (w198:bool[])
                n168 = property on="CurvesInHistogram" class="Arr (strict)"("Value"=w198) -> ()  [unwired: 2 in, 2 out]
                n169 = property on="1-D Histogram?" class="Bool (strict)"("Value"=TRUE ("1-D Histogram?")) -> ()  [unwired: 2 in, 2 out]
                n170 = Select(t=w196, s=w195, f=w200) -> (s? t:f=w203:i32)
                n171 = property on="Continuous?" class="Bool (strict)"("Value"=w195) -> ()  [unwired: 2 in, 2 out]
                n172 = property on="Total 2D Histogram" class="IntGraph (strict)"("Value"=w193) -> ()  [unwired: 2 in, 2 out]
              }
            }
          }
          frame #1 {
            # "Curve Browse:"
            n173 = case shown="True" w208 {
              tunnel: w207 -> [w210 w212]
              tunnel: [w209 w211] -> w206
              frame #0 {
                n174 = Increment(x=w210) -> (x+1=w209:i32)
              }
              frame #1 {
                n175 = Decrement(x=w212) -> (x-1=w211:i32)
              }
            }
            n176 = property on="Continuous?" class="Bool (strict)"("Value"=FALSE ("Continuous?")) -> ()  [unwired: 2 in, 2 out]
          }
        }
      }
    }
  }
